vi "CMD_GOTO.vi"(8 "error in (no error)":errorcluster, 10 "Arguments":string[](array[string]), 11 "gScript Interpreter in":refnum<class "gScript Interpreter.lvclass">) -> (0 "error out":errorcluster, 3 "gScript Interpreter out":refnum<class "gScript Interpreter.lvclass">)   [LabVIEW 2017, in "gScript Interpreter.lvclass"]
uses:
  gScript Interpreter.lvclass
  gScript Interpreter.lvclass/gScript Interpreter.ctl
panel:
  # "Changes the PC to the specified value\n\nExample Uses:\n\n# GOTO a literal command number\nGOTO 10\n\n#GOTO the value stored in a variable\nGOTO $start"
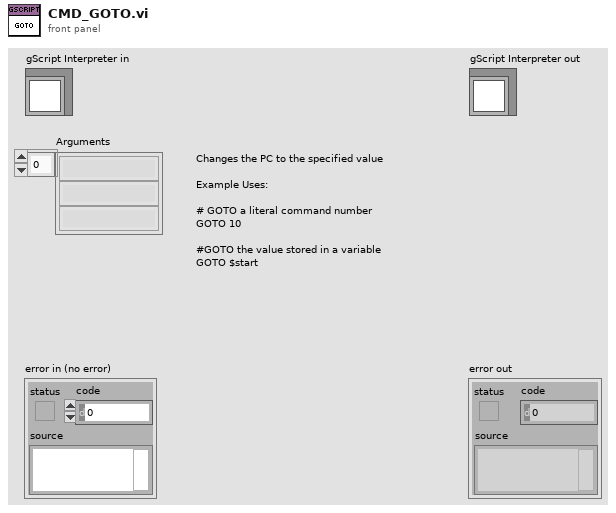
[diagram p1: front panel]
types:
  T1 = typedef "Memory Cell.ctl" = cluster{"type":T2, "x":dbl, "y":dbl, "z":dbl, "w":dbl}
  T2 = typedef "Memory Cell Type Enum.ctl" = enum16{"integer", "float", "vector", "rotation"}
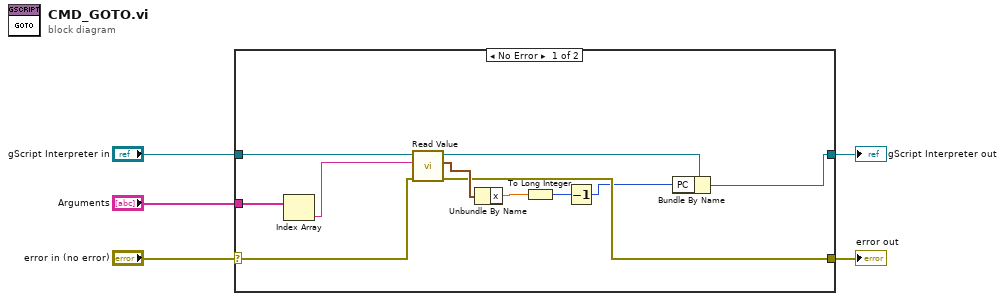
[diagram p0: block diagram]
diagram:
  n1 = case shown="No Error" "error in (no error)" {
    selector: "error in (no error)" -> [w14 w18]
    tunnel: [w11 w18] -> w4
    tunnel: [w6 w17] -> w2
    tunnel: "gScript Interpreter in" -> [w15 w17]
    tunnel: "Arguments" -> [w16 _]
    frame No Error {
      n2 = Index Array(array=w16) -> (element=w13:string)  [unwired: 1 in]
      n3 = call-dynamic "Read Value.vi"("error in (no error)"=w14, "String in"=w13, "gScript Interpreter in"=w15) -> ("error out"=w11:errorcluster, "Memory Cell"=w12:T1, "gScript Interpreter out"=w9:refnum<class "gScript Interpreter.lvclass">)  [unwired: 6 in]
      n4 = Unbundle By Name(w12) -> ("x"=w10:dbl)
      n5 = To Long Integer(number=w10) -> (32bit integer=w8:i32)
      n6 = Decrement(x=w8) -> (x-1=w7:i32)
      n7 = Bundle By Name(cluster=w9, "PC"=w7) -> (w6:refnum<class "gScript Interpreter.lvclass">)
    }
    frame Error {
    }
  }
  "error out" <- w4
  "gScript Interpreter out" <- w2
